vi "test_extractnamesEventRegistrationRefnum.vi"() -> ()   [LabVIEW 2020]
uses:
  _built_ppls/OpenDescriptor.lvlibp
panel:
  out "element names":string[](array[string])
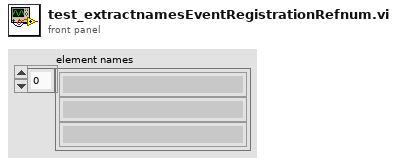
[diagram p1: front panel]
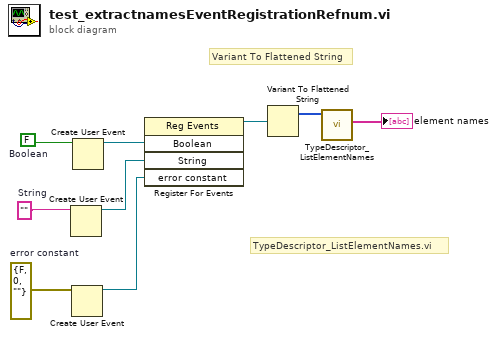
[diagram p0: block diagram]
diagram:
  w2 = errorcluster {"status"=FALSE, "code"=0, "source"=""}  # error constant
  w7 = ""  # String
  w8 = FALSE  # Boolean
  # "Variant To Flattened String"
  # "TypeDescriptor_ListElementNames.vi"
  n1 = Create User Event(user event datatype=w7) -> (user event=w6:refnum<user-event>)  [unwired: 1 in, 1 out]
  n2 = Create User Event(user event datatype=w2) -> (user event=w1:refnum<user-event>)  [unwired: 1 in, 1 out]
  n3 = Create User Event(user event datatype=w8) -> (user event=w9:refnum<user-event>)  [unwired: 1 in, 1 out]
  n4 = register-events(w9, w6, w1) -> (reference out=w5:refnum<event-registration>)  [unwired: 2 in, 1 out]
  n5 = Variant To Flattened String(Variant=w5) -> (1:w4:i16[])  [unwired: 1 out]
  n6 = call "TypeDescriptor_ListElementNames.vi"("type descriptor"=w4) -> ("element names"=→"element names":string[])  [unwired: 7 in, 3 out]
